vi "Read Status.vi"(11 "Test Case Result In":T2) -> (1 "Glyph Index":i32, 2 "Status":T1, 3 "Test Case Result Out":T2)   [LabVIEW 2020, in "Test Case Result.lvlib"]
uses:
  Test Case Result.lvlib
  Test Case Result.ctl
  Method Result/Method Result.ctl
  Assertion Result/Public/TypeDefs/Status.ctl
  Assertion Result/Assertion Result.ctl
  Assertion Result/Public/TypeDefs/Assertion Type.ctl
  Assertion Result/Assertion Result.lvlib
  Method Result/Method Result.lvlib
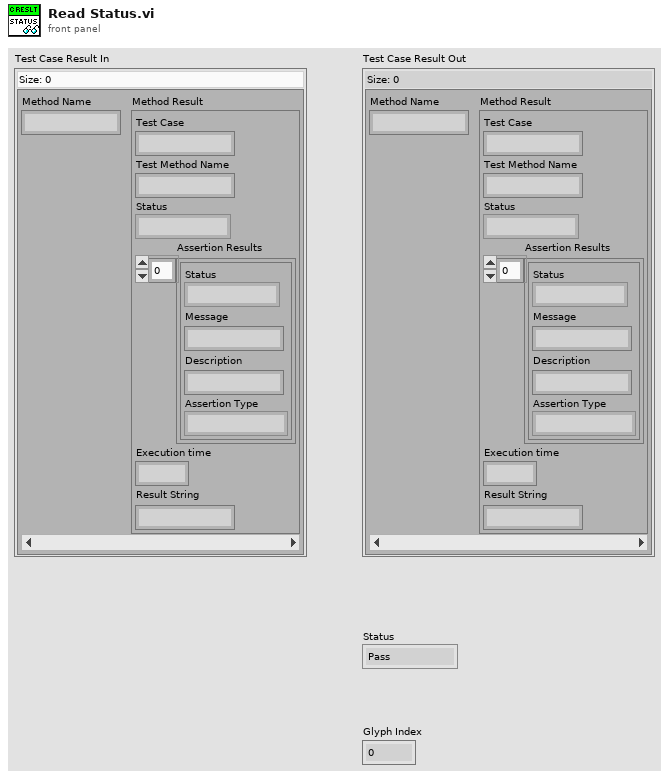
[diagram p1: front panel]
types:
  T1 = typedef "Assertion Result.lvlib/Status.ctl" = enum16{"Pass", "Fail", "Error", "Skipped", "Setup Error", "Broken", "Teardown Error"}
  T2 = typedef "Test Case Result.lvlib/Test Case Result.ctl" = map{string, T3}
  T3 = typedef "Method Result.lvlib/Method Result.ctl" = cluster{"Test Case":string, "Test Method Name":string, "Status":T1, "Assertion Results":T4[], "Execution time":dbl, "Result String":string}
  T4 = typedef "Assertion Result.lvlib/Assertion Result.ctl" = cluster{"Status":T1, "Message":string, "Description":string, "Assertion Type":T5}
  T5 = typedef "Assertion Result.lvlib/Assertion Type.ctl" = enum16{"None", "Pass", "Fail", "Skip", "Pass if Equal", "Fail if Equal", "Pass if Error", "Fail if Error", "Pass if", "Fail if"}
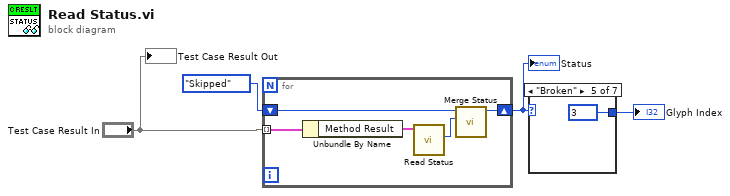
[diagram p0: block diagram]
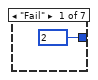
[diagram p2: hidden frame]
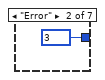
[diagram p3: hidden frame]
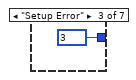
[diagram p4: hidden frame]
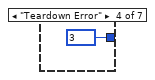
[diagram p5: hidden frame]
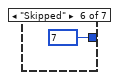
[diagram p6: hidden frame]
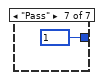
[diagram p7: hidden frame]
diagram:
  n1 = for {
    shift-right: [w7] -> w2
    shift-left: Status."Skipped" ("Status") -> [w9]
    tunnel: "Test Case Result In" -> [w5] mode=indexing
    n2 = Unbundle By Name(w5) -> ("Method Result"=w6:T3)
    n3 = call "Read Status.vi"("Method Result In"=w6) -> ("Status"=w8:T1)  [unwired: 8 in, 2 out]
    n4 = call "Merge Status.vi"("New"=w8, "Current"=w9) -> ("Merged"=w7:T1)  [unwired: 9 in]
  }
  "Status" <- w2
  n5 = case shown="\"Broken\"" w2 {
    tunnel: [2 ("Listbox Symbol Ring Constant") 3 ("Listbox Symbol Ring Constant") 3 ("Listbox Symbol Ring Constant") 3 ("Listbox Symbol Ring Constant") 3 ("Listbox Symbol Ring Constant") 7 ("Listbox Symbol Ring Constant") 1 ("Listbox Symbol Ring Constant")] -> w4
    frame "Fail" {
    }
    frame "Error" {
    }
    frame "Setup Error" {
    }
    frame "Teardown Error" {
    }
    frame "Broken" {
    }
    frame "Skipped" {
    }
    frame "Pass" {
    }
  }
  "Glyph Index" <- w4
  "Test Case Result Out" <- "Test Case Result In"
